vi "Update Frame End Packet Frame ID.vi"(0 "llp packet in":T1, 1 "reset":bool, 9 "input valid":bool, 12 "ready for output":bool) -> (4 "llp packet out":T1, 10 "output valid":bool, 14 "ready for input":bool)   [LabVIEW 2020, in "GettingStarted_Common_148X_FPGA.lvlib"]
uses:
  GettingStarted_Common_148X_FPGA.lvlib
  <instrlib>/FlexRIO/CSI-2/v2/FPGA/Types/LLP Packet.ctl
  <instrlib>/FlexRIO/CSI-2/v2/FPGA/Types/LLP Packet Header.ctl
  <instrlib>/FlexRIO/CSI-2/v2/FPGA/Types/LLP Packet Payload.ctl
  <instrlib>/FlexRIO/CSI-2/v2/FPGA/Types/LLP Packet Footer.ctl
  <instrlib>/_niInstr/Basic Elements/v1/FPGA/Private/Count Up U16.vi
  afc1728f-12c0-4dab-b37c-e4b9395c4be8.vi
  <instrlib>/_niInstr/Basic Elements/v1/FPGA/niInstr Basic Elements v1 FPGA.lvlib
  <instrlib>/FlexRIO/CSI-2/v2/FPGA/NI CSI-2 API FPGA v2.lvlib
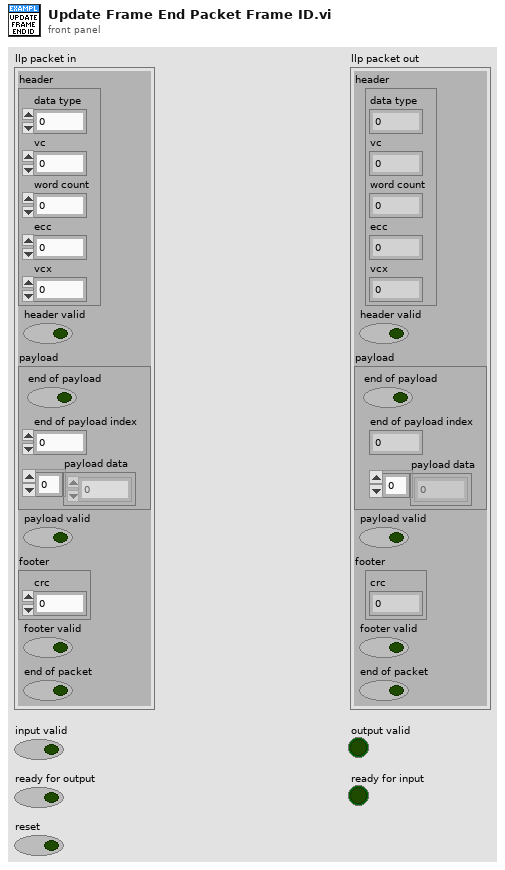
[diagram p1: front panel]
types:
  T1 = typedef "NI CSI-2 API FPGA v2.lvlib/LLP Packet.ctl" = cluster{"header":T2, "header valid":bool, "payload":T3, "payload valid":bool, "footer":T4, "footer valid":bool, "end of packet":bool}
  T2 = typedef "NI CSI-2 API FPGA v2.lvlib/LLP Packet Header.ctl" = cluster{"word count":u16, "ecc":fxp<+,6,6>, "vcx":fxp<+,2,2>, "data type":fxp<+,6,6>, "vc":fxp<+,2,2>}
  T3 = typedef "NI CSI-2 API FPGA v2.lvlib/LLP Packet Payload.ctl" = cluster{"end of payload":bool, "end of payload index":fxp<+,3,3>, "payload data":u8[]}
  T4 = typedef "NI CSI-2 API FPGA v2.lvlib/LLP Packet Footer.ctl" = cluster{"crc":u16}
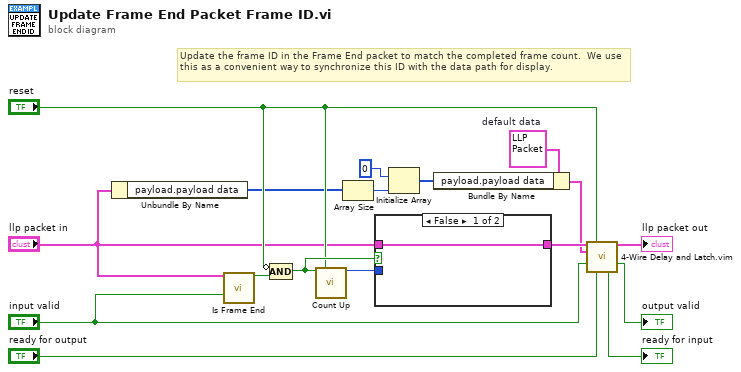
[diagram p0: block diagram]
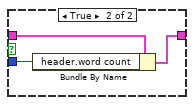
[diagram p2: hidden frame]
diagram:
  w7 = T1 {"header"={"word count"=0, "ecc"=0.0, "vcx"=0.0, "data type"=0.0, "vc"=0.0}, "header valid"=FALSE, "payload"={"end of payload"=FALSE, "end of payload index"=0.0, "payload data"=[]}, "payload valid"=FALSE, "footer"={"crc"=0}, "footer valid"=FALSE, "end of packet"=FALSE}  # default data
  # "Update the frame ID in the Frame End packet to match the completed frame count.  We use this as a convenient way to synchronize this ID with the data path for display."
  n1 = Unbundle By Name("llp packet in") -> ("payload.payload data"=w4:u8[])
  n2 = call <instrlib>:"Is Frame End.vi"("llp packet"="llp packet in", "input valid"="input valid") -> ("frame end"=w17:bool)  [unwired: 13 in]
  n3 = Compound Arithmetic op=AND(invert "reset", w17) -> (w16:bool)
  n4 = call-poly <instrlib>:"Count Up.vi"("increment"=w16, "reset"="reset") -> ("count out"=w15:u16)  [unwired: 13 in]
  n5 = Array Size(array=w4) -> (size(s)=w3:i32)
  n6 = case shown="False" w16 {
    tunnel: "llp packet in" -> [w18 w21]
    tunnel: w15 -> [_ w20]
    tunnel: [w18 w19] -> w13
    frame False {
    }
    frame True {
      n7 = Bundle By Name(cluster=w21, "header.word count"=w20) -> (w19:T1)
    }
  }
  n8 = Initialize Array(u8 0 ("element"), w3) -> (w1:u8[])
  n9 = Bundle By Name(cluster=w7, "payload.payload data"=w1) -> (w6:T1)
  n10 = call "4-Wire Delay and Latch.vim"("data in"=w13, "reset"="reset", "default data"=w6, "input valid"="input valid", "ready for output"="ready for output") -> ("data out"=→"llp packet out":T1, "output valid"=→"output valid":bool, "ready for input"=→"ready for input":bool)  [unwired: 8 in]
